vi "Append LF.vi"(0 "PDF Report IN":refnum<class "PDF Report Class.lvclass">, 1 "Number of LF (default 1)":u8=1, 11 "error in (no error)":errorcluster, 13 "One LF (pts)":sgl=-1.0) -> (4 "PDF Report duplicate":refnum<class "PDF Report Class.lvclass">, 15 "error out":errorcluster)   [LabVIEW 2020, in "Exaprom PDF.lvlib"]
doc: "<B>添加换行符</B>\n向 PDF 报告添加换行符。\nNumber of LF (default 1)----》 换行符（默认1行）\nOne LF（pts）----》默认字体和行距"
uses:
  <userlib>/labview-PDF-writer-master/Exaprom PDF.lvlib
  <userlib>/labview-PDF-writer-master/LV Class/PDF Report Class/PDF Report Class.lvclass
  C:/Program Files (x86)/National Instruments/LabVIEW 2020/user.lib/labview-PDF-writer-master/DLL/itextsharp.dll
  DLL/itextsharp.dll
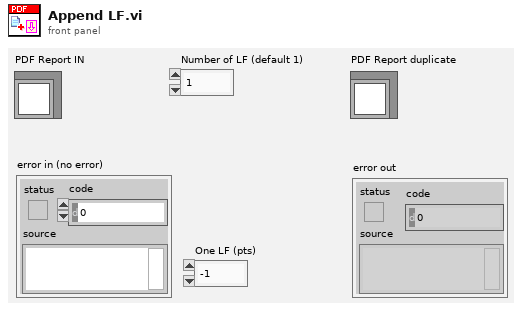
[diagram p1: front panel]
types:
  T1 = typedef "Exaprom PDF.lvlib/Font size.ctl" = sgl
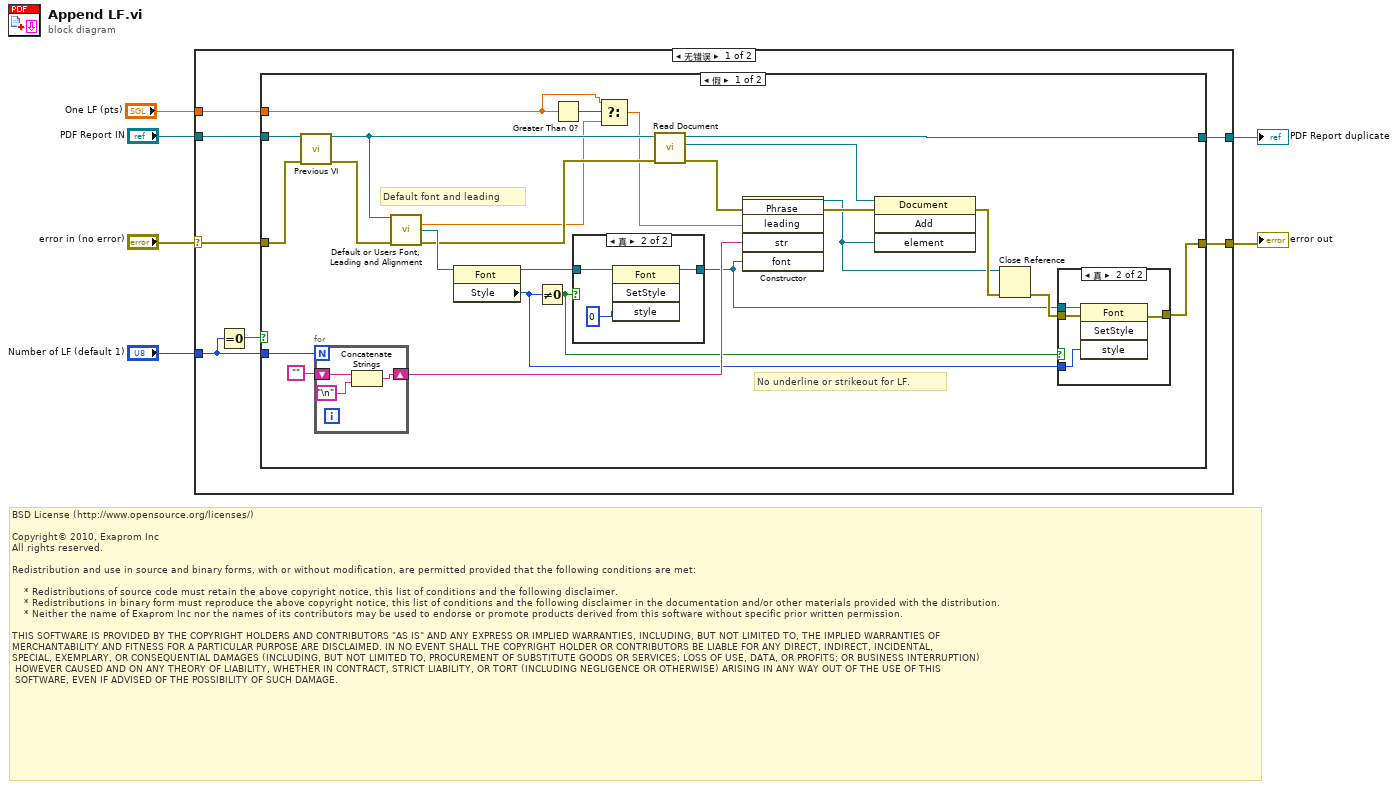
[diagram p0: block diagram]
diagram:
  # "BSD License (http://www.opensource.org/licenses/)\n\nCopyright© 2010, Exaprom Inc\nAll rights reserved.\n\nRedistribution and use in source and binary forms, with or without modification, are permitted provided that the following conditions are met:\n\n    * Redistributions of source code must retain the above copyright notice, this list of conditions and the following disclaimer.\n    * Redistributions in binary form must reproduce the above copyright notice, this list of conditions and the following disclaimer in the documentation and/or other materials provided with the distribution.\n    * Neither the name of Exaprom Inc nor the names of its contributors may be used to endorse or promote products derived from this software without specific prior written permission.\n\nTHIS SOFTWARE IS PROVIDED BY THE COPYRIGHT HOLDERS AND CONTRIBUTORS \"AS IS\" AND ANY EXPRESS OR IMPLIED WARRANTIES, INCLUDING, BUT NOT LIMITED TO, THE IMPLIED WARRANTIES OF \nMERCHANTABILITY AND FITNESS FOR A PARTICULAR PURPOSE ARE DISCLAIMED. IN NO EVENT SHALL THE COPYRIGHT HOLDER OR CONTRIBUTORS BE LIABLE FOR ANY DIRECT, INDIRECT, INCIDENTAL,\nSPECIAL, EXEMPLARY, OR CONSEQUENTIAL DAMAGES (INCLUDING, BUT NOT LIMITED TO, PROCUREMENT OF SUBSTITUTE GOODS OR SERVICES; LOSS OF USE, DATA, OR PROFITS; OR BUSINESS INTERRUPTION)\n HOWEVER CAUSED AND ON ANY THEORY OF LIABILITY, WHETHER IN CONTRACT, STRICT LIABILITY, OR TORT (INCLUDING NEGLIGENCE OR OTHERWISE) ARISING IN ANY WAY OUT OF THE USE OF THIS\n SOFTWARE, EVEN IF ADVISED OF THE POSSIBILITY OF SUCH DAMAGE."
  n1 = case shown="无错误" "error in (no error)" {
    selector: "error in (no error)" -> [w12 w54]
    tunnel: [w13 w53] -> w3
    tunnel: [w10 w54] -> w6
    tunnel: "PDF Report IN" -> [w11 w53]
    tunnel: "Number of LF (default 1)" -> [w9 _]
    tunnel: "One LF (pts)" -> [w7 _]
    frame No Error {
      n2 = Equal To 0?(x=w9) -> (x = 0?=w8:bool)
      n3 = case shown="假" w8 {
        tunnel: [w22 w52] -> w13
        tunnel: w12 -> [w38 w51]
        tunnel: w11 -> [w33 w52]
        tunnel: [w31 w51] -> w10
        tunnel: w9 -> [w27 _]
        tunnel: w7 -> [w16 _]
        frame False {
          # "Default font and leading"
          # "No underline or strikeout for LF."
          n4 = call <userlib>:"Previous VI.vi"("PDF Report IN"=w33, "error in (no error)"=w38) -> ("PDF Report OUT"=w18:refnum<class "PDF Report Class.lvclass">, "error out"=w37:errorcluster)  [unwired: 12 out]
          n5 = for {
            N: w27 -> [_]
            shift-right: [w45] -> w26
            shift-left: "" -> [w44]
            n6 = Concatenate Strings(w44, "\n") -> (w45:string)
          }
          n7 = call <userlib>:"Default or Users Font, Leading and Alignment.vi"("PDF Report"=w18, "error in (no error)"=w37) -> ("Leading"=w15:T1, "Font Ref"=w30:refnum<k24>, "error out"=w20:errorcluster)  [unwired: 2 in, 9 out]
          n8 = property class="Font"(reference=w30) -> (reference out=w29:refnum<k24>, "Style"=w24:i32)  [unwired: 1 in, 1 out]
          n9 = Not Equal To 0?(x=w24) -> (x != 0?=w23:bool)
          n10 = Greater Than 0?(x=w16) -> (x > 0?=w17:bool)
          n11 = case shown="真" w23 {
            tunnel: w29 -> [w39 w41]
            tunnel: [w39 w40] -> w25
            frame False {
            }
            frame True {
              n12 = invoke class="Font" method="SetStyle"(reference=w41, "style"=0) -> (reference out=w40:refnum<k24>)  [unwired: 2 in, 3 out]
            }
          }
          n13 = Select(t=w16, s=w17, f=w15) -> (s? t:f=w14:T1)
          n14 = call-dynamic "Read Document.vi"("error in (no error)"=w20, "PDF Report Class in"=w18) -> ("error out"=w19:errorcluster, "Document"=w21:refnum<k24>, "PDF Report Class out"=w22:refnum<class "PDF Report Class.lvclass">)  [unwired: 7 in]
          n15 = constructor class="Phrase"(error in=w19, "leading"=w14, "str"=w26, "font"=w25) -> (reference out=w34:refnum<k24>, error out=w35:errorcluster)  [unwired: 2 in, 4 out]
          n16 = invoke class="Document" method="Add"(reference=w21, error in=w35, "element"=w34) -> (error out=w36:errorcluster)  [unwired: 1 in, 3 out]
          n17 = Close Reference(reference=w34, error in (no error)=w36) -> (error out=w32:errorcluster)
          n18 = case shown="真" w23 {
            tunnel: w32 -> [w46 w50]
            tunnel: [w46 w49] -> w31
            tunnel: w24 -> [_ w48]
            tunnel: w25 -> [_ w47]
            frame False {
            }
            frame True {
              n19 = invoke class="Font" method="SetStyle"(reference=w47, error in=w50, "style"=w48) -> (error out=w49:errorcluster)  [unwired: 1 in, 3 out]
            }
          }
        }
        frame True {
        }
      }
    }
    frame Error {
    }
  }
  "error out" <- w6
  "PDF Report duplicate" <- w3
